vi "libssh2_knownhost_addc.vi"(4 "comment":string, 6 "salt":string, 7 "typemask":T2 items=["TYPE_PLAIN"=1, "TYPE_SHA1"=2, "TYPE_CUSTOM"=3, "KEYENC_RAW"=65536, "KEYENC_BASE64"=131072, "KEY_RSA1"=262144, "KEY_SSHRSA"=524288, "KEY_SSHDSS"=786432, "KEY_ECDSA_256"=1048576, "KEY_ECDSA_384"=1310720, "KEY_ECDSA_521"=1572864, "KEY_ED25519"=1835008, "KEY_UNKNOWN"=3932160], 8 "error in (no error)":errorcluster, 9 "key":u8[](array[numeric]), 10 "hostname":string, 11 "host key database":T3) -> (0 "error out":errorcluster, 3 "host key":T1)   [LabVIEW 2013, in "libssh2.lvlib"]
doc: "Add a host key to a host key database."
uses:
  libssh2.lvlib
  Host Key Database Refnum.ctl
  libssh2_knownhost_typemask.ctl
  Host Key Refnum.ctl
  Not A Host Key Database.vi
  <vilib>/Utility/error.llb/Error Cluster From Error Code.vi
  Global Settings.vi
  Read Host Key Database Refnum.vi
  <vilib>/Utility/semaphor.llb/Acquire Semaphore.vi
  <vilib>/Utility/semaphor.llb/Release Semaphore.vi
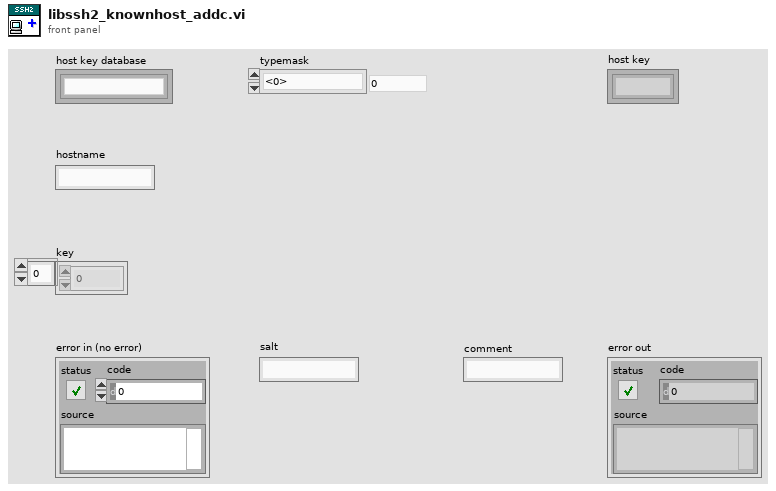
[diagram p1: front panel]
types:
  T1 = typedef "libssh2.lvlib/Host Key Refnum.ctl" = refnum<k1>
  T2 = typedef "libssh2.lvlib/libssh2_knownhost_typemask.ctl" = i32
  T3 = typedef "libssh2.lvlib/Host Key Database Refnum.ctl" = refnum<k1>
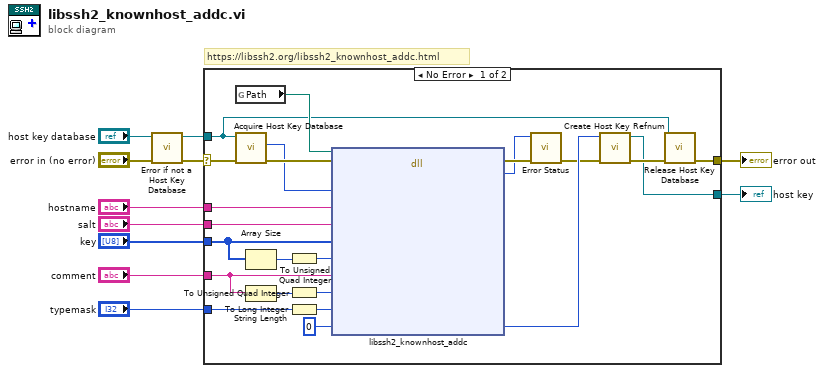
[diagram p0: block diagram]
diagram:
  # "https://libssh2.org/libssh2_knownhost_addc.html"
  n1 = call "Error if not a Host Key Database.vi"("error in (no error)"="error in (no error)", "host key database"="host key database") -> ("error out"=w9:errorcluster, "host key database out"=w7:T3)  [unwired: 8 in]
  n2 = case shown="No Error" w9 {
    selector: w9 -> [w32 w35]
    tunnel: [w13 w35] -> w11
    tunnel: w7 -> [w12 _]
    tunnel: [w33 _] -> w6
    tunnel: "typemask" -> [w23 _]
    tunnel: "comment" -> [w17 _]
    tunnel: "key" -> [w19 _]
    tunnel: "salt" -> [w22 _]
    tunnel: "hostname" -> [w21 _]
    frame No Error {
      n3 = global read "Global Settings.vi" "Path"() -> (w27:path)
      n4 = call "Acquire Host Key Database.vi"("error in (no error)"=w32, "host key database"=w12) -> ("error out"=w30:errorcluster, "LIBSSH2_KNOWNHOSTS*"=w29:u64)  [unwired: 8 in]
      n5 = Array Size(array=w19) -> (size(s)=w20:i32)
      n6 = String Length(string=w17) -> (length=w18:i32)
      n7 = To Unsigned Quad Integer(1:w20) -> (0:w16:u64)
      n8 = To Unsigned Quad Integer(1:w18) -> (0:w15:u64)
      n9 = To Long Integer(number=w23) -> (32bit integer=w14:T2)
      n10 = dll-call lib="?" fn="libssh2_knownhost_addc"(path in=w27, error in=w30, "hosts"=w29, "host"=w21, "salt"=w22, "key"=w19, "keylen"=w16, "comment"=w17, "commentlen"=w15, "typemask"=w14, "store"=u64 0) -> (error out=w31:errorcluster, "return value"=w25:i32, "store"=w28:u64)  [unwired: 9 in, 1 out]
      n11 = call "Error Status.vi"("error in (no error)"=w31, "return value"=w25) -> ("error out"=w26:errorcluster)  [unwired: 8 in, 1 out]
      n12 = call "Create Host Key Refnum.vi"("error in (no error)"=w26, "libssh2_knownhost*"=w28) -> ("error out"=w34:errorcluster, "host key"=w33:T1)  [unwired: 8 in]
      n13 = call "Release Host Key Database.vi"("error in (no error)"=w34, "host key database"=w12) -> ("error out"=w13:errorcluster)  [unwired: 9 in]
    }
    frame Error {
    }
  }
  "error out" <- w11
  "host key" <- w6
